vi "Request Data JSON.vi"(8 "error in (no error)":errorcluster, 11 "JSONRequest in":refnum<class "JSONRequest.lvclass">) -> (0 "error out":errorcluster, 2 "Request Data JSON":string, 3 "JSONRequest out":refnum<class "JSONRequest.lvclass">)   [LabVIEW 2020, in "obs-websocket.lvlib" / "JSONRequest.lvclass"]
uses:
  JSONRequest.lvclass
  JSONRequest.lvclass/JSONRequest.ctl
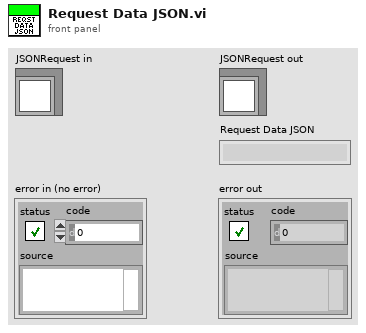
[diagram p1: front panel]
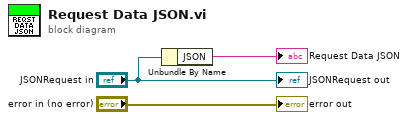
[diagram p0: block diagram]
diagram:
  n1 = Unbundle By Name("JSONRequest in") -> ("JSON"=→"Request Data JSON":string)
  "error out" <- "error in (no error)"
  "JSONRequest out" <- "JSONRequest in"
